vi "PH_Beckhoff_PP_Control.set i Attr and start DIM Services.vi"(0 "i ref in":refnum<vi>, 2 "Values":T6, 5 "error in":errorcluster) -> (14 "i ref out":refnum<vi>, 17 "i Attr":T1={"PP Conductivity Control"={"PSDB"={"Status Service ID"=-1, "Instance ID"=-1, "Data Status"=0, "Ref Status"=refnum, "Error Code"=0}, "Status"={"GUI Ref"=refnum, "Status Service ID"=-1, "Status"=0}, "DIs"={"Device on"={"GUI Ref"=refnum, "# in Data"=-1}, "Conductivity ok"={"GUI Ref"=refnum, "# in Data"=-1}, "Temperature ok"={"GUI Ref"=refnum, "# in Data"=-1}, "Alarm"={"GUI Ref"=refnum, "# in Data"=-1}}, "PSDB Thread"={"Ref"=refnum, "Q-Ref"=refnum}}, "PP Mercury Control"={"PSDB"={"Status Service ID"=-1, "Instance ID"=-1, "Data Status"=0, "Ref Status"=refnum, "Error Code"=0}, "Status"={"GUI Ref"=refnum, "Status Service ID"=-1, "Status"=0}, "on since:"={"GUI Ref"=refnum, "Service ID"=-1, "Time"=""}, "DIs"={"Device on"={"GUI Ref"=refnum, "# in Data"=-1}, "Alarm"={"GUI Ref"=refnum, "# in Data"=-1}}, "AIs"={"Concentration"={"GUI Ref"=refnum, "# in Data"=-1}}, "PSDB Thread"={"Ref"=refnum, "Q-Ref"=refnum}}, "PSDB"={"Shot #"=-1, "Subsystem"=0}, "PSDB Credentials"={"PW"="N/A", "ID"="N/A", "DS"="N/A"}} {"PSDB"."Subsystem" items=["Miscellaneous", "fs-Frontend", "ns-Frontend", "PreAmp", "MainAmp", "MAS", "COS", "Beamline", "Experiment Laserbay", "Experiment Laserlabor", "Experiment Z6", "Timing", "Pulsed Power"]; "PP Mercury Control"."Status"."Status" items=["no info", "off/false/out", "on/true/in", "Failure", "Alarm", "Status 1", "Status 2", "Status 3"]; "PP Mercury Control"."PSDB"."Data Status" items=["no info", "no Data collection", "no problem", "Error getting the ID", "Error writing Data", "Error getting the subsystem", "Error getting the Shot ID", "Error getting the Shot Types", "Error getting the Experiments", "Error verifying wanted Shottype", "Error verifying wanted Experiment"]; "PP Conductivity Control"."Status"."Status" items=["no info", "off/false/out", "on/true/in", "Failure", "Alarm", "Status 1", "Status 2", "Status 3"]; "PP Conductivity Control"."PSDB"."Data Status" items=["no info", "no Data collection", "no problem", "Error getting the ID", "Error writing Data", "Error getting the subsystem", "Error getting the Shot ID", "Error getting the Shot Types", "Error getting the Experiments", "Error verifying wanted Shottype", "Error verifying wanted Experiment"]}, 19 "error out":errorcluster)   [LabVIEW 2014, in "PH_Beckhoff_PP_Control.lvlib"]
doc: "This VI gets the # of relevant data in the related data array(s) and stores them at own attributes."
uses:
  PH_Beckhoff_PP_Control.lvlib
  PH_Beckhoff/PH_Beckhoff.Values.ctl
  PH_Beckhoff/PH_Beckhoff.Sonderklemmen Inputs.ctl
  PH_Beckhoff/PH_Beckhoff.Analog Inputs.ctl
  PH_Beckhoff/PH_Beckhoff.Scaling Type.ctl
  PH_Beckhoff/PH_Beckhoff.Analog Outputs.ctl
  PH_Beckhoff/PH_Beckhoff.Digital Inputs.ctl
  PH_Beckhoff/PH_Beckhoff.Digital Outputs.ctl
  PH_Beckhoff_PP_Control.i attribute.ctl
  PH_PSDBWriter/PH_PSDBWriter.Data Status.ctl
  PH_StatusHandler/PH_StatusHandler.Status.ctl
  PH_PSDBWriter/PH_PSDBWriter.PHELIX-Subsystems.ctl
  PH_Common/Connection/PH_Connection.PSDB Credentials.ctl
  PH_Beckhoff_PP_Control.PP Conductivity Tags.ctl
  PH_Beckhoff_PP_Control.PP Mercury Tags.ctl
  PH_PSDBWriter/PH_PSDBWriter.lvlib
  PH_StatusHandler/PH_StatusHandler.lvlib
  lib.lib/DimLVEvent/LVDimInterface/LVDimInterface.lvlib
  lib.lib/UtilityLib/UtilityLib.lvlib
  CSCore/CSSystem/CSSystemLib/CSSystemLib.lvlib
  PH_Common/PH_Common.lvlib
  PH_Beckhoff/PH_Beckhoff.lvlib
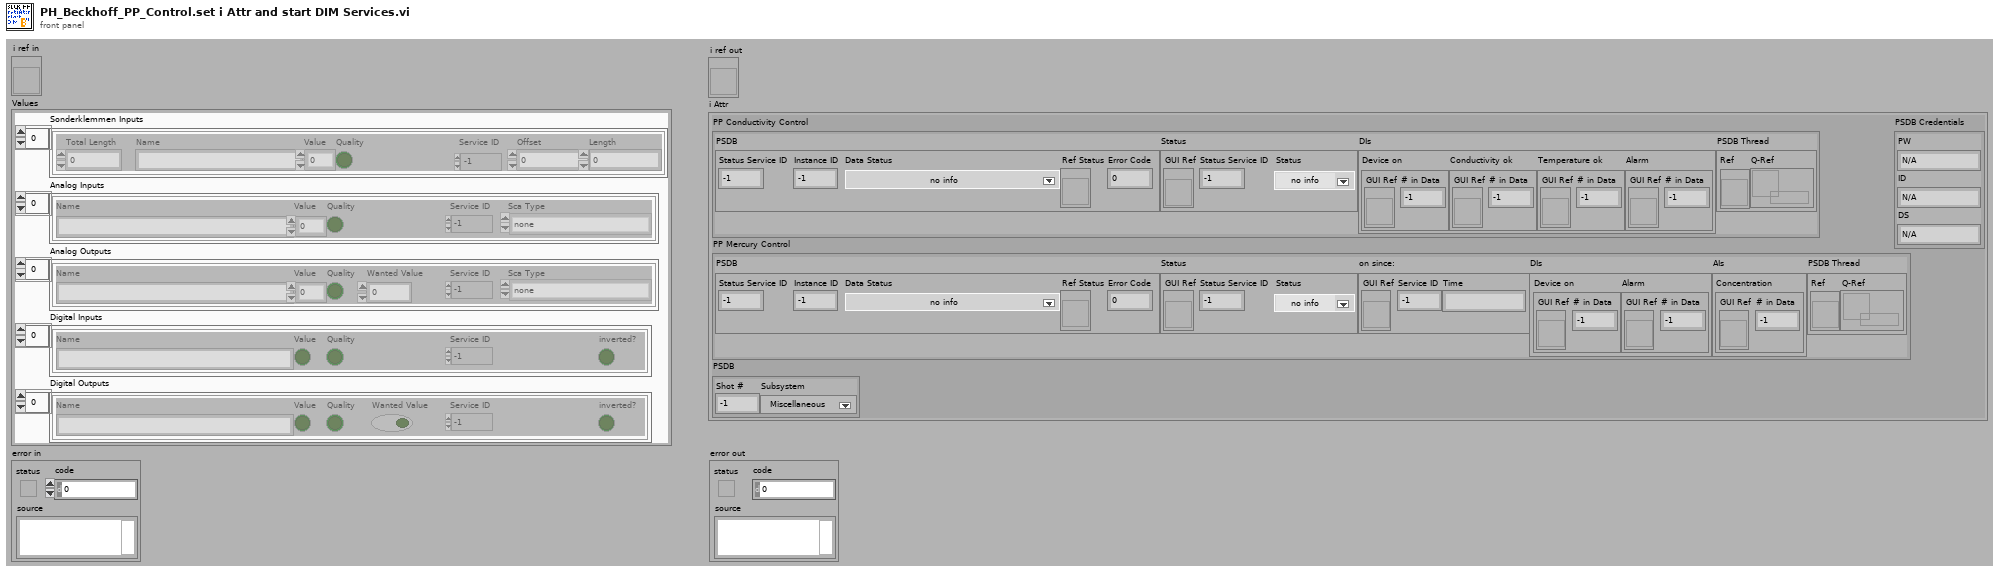
[diagram p1: front panel]
types:
  T1 = typedef "PH_Beckhoff_PP_Control.lvlib/PH_Beckhoff_PP_Control.i attribute.ctl" = cluster{"PP Conductivity Control":cluster{"PSDB":cluster{"Status Service ID":i32, "Instance ID":i32, "Data Status":T2, "Ref Status":refnum<vi>, "Error Code":i32}, "Status":cluster{"GUI Ref":refnum<vi>, "Status Service ID":i32, "Status":T3}, "DIs":cluster{"Device on":cluster{"GUI Ref":refnum<vi>, "# in Data":i32}, "Conductivity ok":cluster{"GUI Ref":refnum<vi>, "# in Data":i32}, "Temperature ok":cluster{"GUI Ref":refnum<vi>, "# in Data":i32}, "Alarm":cluster{"GUI Ref":refnum<vi>, "# in Data":i32}}, "PSDB Thread":cluster{"Ref":refnum<vi>, "Q-Ref":refnum<queue>}}, "PP Mercury Control":cluster{"PSDB":cluster{"Status Service ID":i32, "Instance ID":i32, "Data Status":T2, "Ref Status":refnum<vi>, "Error Code":i32}, "Status":cluster{"GUI Ref":refnum<vi>, "Status Service ID":i32, "Status":T3}, "on since:":cluster{"GUI Ref":refnum<vi>, "Service ID":i32, "Time":string}, "DIs":cluster{"Device on":cluster{"GUI Ref":refnum<vi>, "# in Data":i32}, "Alarm":cluster{"GUI Ref":refnum<vi>, "# in Data":i32}}, "AIs":cluster{"Concentration":cluster{"GUI Ref":refnum<vi>, "# in Data":i32}}, "PSDB Thread":cluster{"Ref":refnum<vi>, "Q-Ref":refnum<queue>}}, "PSDB":cluster{"Shot #":i32, "Subsystem":T4}, "PSDB Credentials":T5}
  T2 = typedef "PH_PSDBWriter.lvlib/PH_PSDBWriter.Data Status.ctl" = i16
  T3 = typedef "PH_StatusHandler.lvlib/PH_StatusHandler.Status.ctl" = i16
  T4 = typedef "PH_PSDBWriter.lvlib/PH_PSDBWriter.PHELIX-Subsystems.ctl" = i32
  T5 = typedef "PH_Common.lvlib/PH_Connection.PSDB Credentials.ctl" = cluster{"PW":string, "ID":string, "DS":string}
  T6 = typedef "PH_Beckhoff.lvlib/PH_Beckhoff.Values.ctl" = cluster{"Sonderklemmen Inputs":T7, "Analog Inputs":T8, "Analog Outputs":T10, "Digital Inputs":T11, "Digital Outputs":T12}
  T7 = typedef "PH_Beckhoff.lvlib/PH_Beckhoff.Sonderklemmen Inputs.ctl" = cluster{"Total Length":u32, "Name":string, "Value":u64, "Quality":bool, "Service ID":i32, "Offset":u32, "Length":u32}[]
  T8 = typedef "PH_Beckhoff.lvlib/PH_Beckhoff.Analog Inputs.ctl" = cluster{"Name":string, "Value":u32, "Quality":bool, "Service ID":i32, "Sca Type":T9}[]
  T9 = typedef "PH_Beckhoff.lvlib/PH_Beckhoff.Scaling Type.ctl" = enum16{"none", "0 ... 15 Bit -> 0 ... 5", "0 ... 15 Bit -> 0 ... 10", "0 ... 15 Bit -> 0 ... 25", "0 ... 15 Bit -> 4 ... 20", "0 ... 15 Bit -> 0 ... 1", "0 ... 15 Bit -> 0 ... 20000", "0 ... 15 Bit -> 0 ... 24000"}
  T10 = typedef "PH_Beckhoff.lvlib/PH_Beckhoff.Analog Outputs.ctl" = cluster{"Name":string, "Value":u32, "Quality":bool, "Wanted Value":u32, "Service ID":i32, "Sca Type":T9}[]
  T11 = typedef "PH_Beckhoff.lvlib/PH_Beckhoff.Digital Inputs.ctl" = cluster{"Name":string, "Value":bool, "Quality":bool, "Service ID":i32, "inverted?":bool}[]
  T12 = typedef "PH_Beckhoff.lvlib/PH_Beckhoff.Digital Outputs.ctl" = cluster{"Name":string, "Value":bool, "Quality":bool, "Wanted Value":bool, "Service ID":i32, "inverted?":bool}[]
  T13 = typedef "PH_Beckhoff_PP_Control.lvlib/PH_Beckhoff_PP_Control.PP Mercury Tags.ctl" = enum16{"Device-on", "Alarm", "on-since", "Concentration", "Status"}
  T14 = typedef "PH_Beckhoff_PP_Control.lvlib/PH_Beckhoff_PP_Control.PP Conductivity Tags.ctl" = enum16{"Device-on", "Conductivity-2-high", "Temperature-not-2-low", "Alarm", "Conductivity", "Status"}
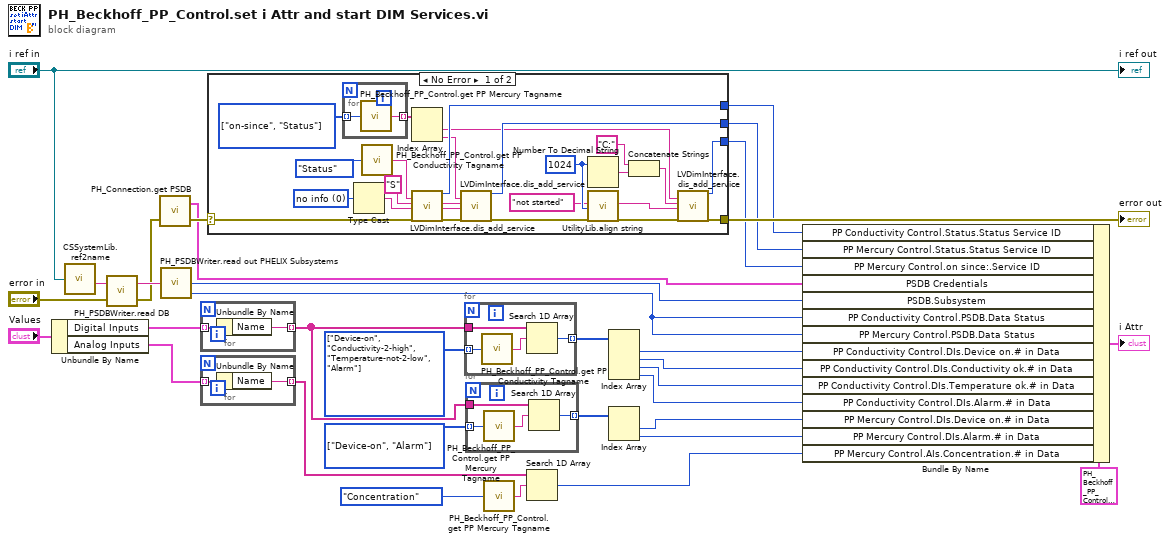
[diagram p0: block diagram]
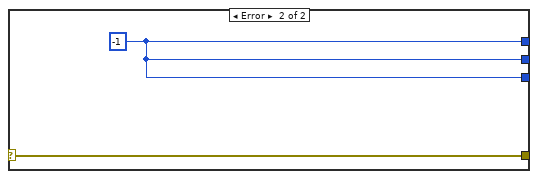
[diagram p2: hidden frame]
diagram:
  w29 = T13[] [enum."Device-on", enum."Alarm"] items=["Device-on", "Alarm", "on-since", "Concentration", "Status"]
  w30 = T14[] [enum."Device-on", enum."Conductivity-2-high", enum."Temperature-not-2-low", enum."Alarm"] items=["Device-on", "Conductivity-2-high", "Temperature-not-2-low", "Alarm", "Conductivity", "Status"]
  n1 = Unbundle By Name("Values") -> ("Digital Inputs"=w33:T11, "Analog Inputs"=w25:T8)
  n2 = call "CSSystemLib.ref2name.vi"("obj refnum"="i ref in") -> ("name"=w4:string)
  n3 = call "PH_PSDBWriter.read DB.vi"("error in"="error in", "Instance Name"=w4) -> ("error out"=w3:errorcluster, "PSDB Subsystem"=w13:string)
  n4 = call "PH_Connection.get PSDB.vi"("error in (no error)"=w3) -> ("error out"=w2:errorcluster, "PSDB Credentials"=w1:T5)  [unwired: 1 in]
  n5 = call "PH_PSDBWriter.read out PHELIX Subsystems.vi"("Config DB Subsystem"=w13) -> ("Metadata.Data Status"=w11:T2, "Metadata.Subsystem"=w10:T4)  [unwired: 2 in, 1 out]
  n6 = for {
    tunnel: w33 -> [w35] mode=indexing
    tunnel: [w34] -> w27 mode=indexing
    n7 = Unbundle By Name(w35) -> ("Name"=w34:string)
  }
  n8 = for {
    tunnel: w25 -> [w37] mode=indexing
    tunnel: [w36] -> w24 mode=indexing
    n9 = Unbundle By Name(w37) -> ("Name"=w36:string)
  }
  n10 = case shown="No Error" w2 {
    selector: w2 -> [w59 w64]
    tunnel: [w60 w63] -> w6
    tunnel: [w38 w64] -> w9
    tunnel: [w51 w63] -> w7
    tunnel: [w40 w63] -> w8
    frame No Error {
      w43 = u16 1024 ("String Length (1024)")
      w50 = T13[] [enum."on-since", enum."Status"] items=["Device-on", "Alarm", "on-since", "Concentration", "Status"]
      w57 = T3 0 items=["no info", "off/false/out", "on/true/in", "Failure", "Alarm", "Status 1", "Status 2", "Status 3"] ("Status")
      w55 = "S" ("typeDescriptor")
      n11 = for {
        tunnel: [w62] -> w53 mode=indexing
        tunnel: w50 -> [w61] mode=indexing
        n12 = call "PH_Beckhoff_PP_Control.get PP Mercury Tagname.vi"("PP Mercury Tag"=w61) -> ("PP Mercury Tagname"=w62:string)
      }
      n13 = Type Cast(x=w57) -> (*(type *) &x=w54:string)  [unwired: 1 in]
      n14 = call "PH_Beckhoff_PP_Control.get PP Conductivity Tagname.vi"("PP Conductivity Tag"=PH_Beckhoff_PP_Control.PP_Conductivity_Tags."Status") -> ("PP Conductivity Tagname"=w58:string)
      n15 = Index Array(array=w53) -> (element #1=w41:string, element #2=w49:string)  [unwired: 2 in]
      n16 = call "LVDimInterface.dis_add_service.vi"("serviceName"=w58, "typeDescriptor"=w55, "data"=w54, "error in (no error)"=w59) -> ("my_serviceID"=w60:i32, "error out"=w52:errorcluster)  [unwired: 14 in]
      n17 = call "LVDimInterface.dis_add_service.vi"("serviceName"=w49, "typeDescriptor"=w55, "data"=w54, "error in (no error)"=w52) -> ("my_serviceID"=w51:i32, "error out"=w39:errorcluster)  [unwired: 14 in]
      n18 = Number To Decimal String(number=w43) -> (decimal integer string=w48:string)  [unwired: 1 in]
      n19 = call "UtilityLib.align string.vi"("stringIn"="not started" ("String"), "stringLength (80)"=w43, "error in (no error)"=w39) -> ("stringOut"=w44:string, "error out"=w45:errorcluster)  [unwired: 15 in]
      n20 = Concatenate Strings("C:" ("typeDescriptor"), w48) -> (w47:string)
      n21 = call "LVDimInterface.dis_add_service.vi"("serviceName"=w41, "typeDescriptor"=w47, "data"=w44, "error in (no error)"=w45) -> ("my_serviceID"=w40:i32, "error out"=w38:errorcluster)  [unwired: 14 in]
    }
    frame Error {
      w63 = -1 ("my_serviceID")
    }
  }
  "error out" <- w9
  n22 = for {
    tunnel: w30 -> [w68] mode=indexing
    tunnel: w27 -> [w67]
    tunnel: [w65] -> w31 mode=indexing
    n23 = call "PH_Beckhoff_PP_Control.get PP Conductivity Tagname.vi"("PP Conductivity Tag"=w68) -> ("PP Conductivity Tagname"=w66:string)
    n24 = Search 1D Array(1D array=w67, element=w66) -> (index of element=w65:i32)  [unwired: 1 in]
  }
  n25 = for {
    tunnel: w27 -> [w72]
    tunnel: [w70] -> w28 mode=indexing
    tunnel: w29 -> [w69] mode=indexing
    n26 = call "PH_Beckhoff_PP_Control.get PP Mercury Tagname.vi"("PP Mercury Tag"=w69) -> ("PP Mercury Tagname"=w71:string)
    n27 = Search 1D Array(1D array=w72, element=w71) -> (index of element=w70:i32)  [unwired: 1 in]
  }
  n28 = call "PH_Beckhoff_PP_Control.get PP Mercury Tagname.vi"("PP Mercury Tag"=PH_Beckhoff_PP_Control.PP_Mercury_Tags."Concentration") -> ("PP Mercury Tagname"=w23:string)
  n29 = Search 1D Array(1D array=w24, element=w23) -> (index of element=w22:i32)  [unwired: 1 in]
  n30 = Index Array(array=w31) -> (element #1=w21:i32, element #2=w20:i32, element #3=w19:i32, element #4=w18:i32)  [unwired: 4 in]
  n31 = Index Array(array=w28) -> (element #1=w17:i32, element #2=w16:i32)  [unwired: 2 in]
  n32 = Bundle By Name(cluster=T1 {"PP Conductivity Control"={"PSDB"={"Status Service ID"=-1, "Instance ID"=-1, "Data Status"=0, "Ref Status"=refnum, "Error Code"=0}, "Status"={"GUI Ref"=refnum, "Status Service ID"=-1, "Status"=0}, "DIs"={"Device on"={"GUI Ref"=refnum, "# in Data"=-1}, "Conductivity ok"={"GUI Ref"=refnum, "# in Data"=-1}, "Temperature ok"={"GUI Ref"=refnum, "# in Data"=-1}, "Alarm"={"GUI Ref"=refnum, "# in Data"=-1}}, "PSDB Thread"={"Ref"=refnum, "Q-Ref"=refnum}}, "PP Mercury Control"={"PSDB"={"Status Service ID"=-1, "Instance ID"=-1, "Data Status"=0, "Ref Status"=refnum, "Error Code"=0}, "Status"={"GUI Ref"=refnum, "Status Service ID"=-1, "Status"=0}, "on since:"={"GUI Ref"=refnum, "Service ID"=-1, "Time"=""}, "DIs"={"Device on"={"GUI Ref"=refnum, "# in Data"=-1}, "Alarm"={"GUI Ref"=refnum, "# in Data"=-1}}, "AIs"={"Concentration"={"GUI Ref"=refnum, "# in Data"=-1}}, "PSDB Thread"={"Ref"=refnum, "Q-Ref"=refnum}}, "PSDB"={"Shot #"=-1, "Subsystem"=0}, "PSDB Credentials"={"PW"="N/A", "ID"="N/A", "DS"="N/A"}} ("i attribute"), "PP Conductivity Control.Status.Status Service ID"=w6, "PP Mercury Control.Status.Status Service ID"=w7, "PP Mercury Control.on since:.Service ID"=w8, "PSDB Credentials"=w1, "PSDB.Subsystem"=w10, "PP Conductivity Control.PSDB.Data Status"=w11, "PP Mercury Control.PSDB.Data Status"=w11, "PP Conductivity Control.DIs.Device on.# in Data"=w21, "PP Conductivity Control.DIs.Conductivity ok.# in Data"=w20, "PP Conductivity Control.DIs.Temperature ok.# in Data"=w19, "PP Conductivity Control.DIs.Alarm.# in Data"=w18, "PP Mercury Control.DIs.Device on.# in Data"=w17, "PP Mercury Control.DIs.Alarm.# in Data"=w16, "PP Mercury Control.AIs.Concentration.# in Data"=w22) -> (→"i Attr":T1)
  "i ref out" <- "i ref in"
